vi "Test.vi"() -> ()   [LabVIEW 2015, in "LabSSH.lvlib"]
doc: "<License>This software is distributed under the BSD 3-Clause License. For the full license please see license.txt or visit www.labvolution.com/license</License>"
uses:
  LabSSH.lvlib
  Connection Info..cluster.ctl
  Password..cluster.ctl
  Private Public Key..cluster.ctl
  <vilib>/Utility/miscctls.llb/LVForegroundBackgroundColorsTypeDef.ctl
  connect_password.vi
  connect_key.vi
panel:
  in  "Connection Name":string
  in  "Close":bool
  in  "Connect":bool
  in  "Expected Response":string
  in  "Private_Public Key":T1
  in  "Connection Type":enum16{"Password", "Private Key"}(ring)
  out "Method Response":string
  in  "error in (no error)":errorcluster
  out "isSshConnected":bool
  in  "Password":T2
  in  "Connection Info.":T3={"Remote"="", "Username"="", "Port (22)"=22}
  out "Output":string
  # "http://www.labvolution.com/blog/"
  # "C:\\\\Working Folder\\\\ssh.git\\\\LabSSH\\\\raspberrypi_private_openssh.ppk"
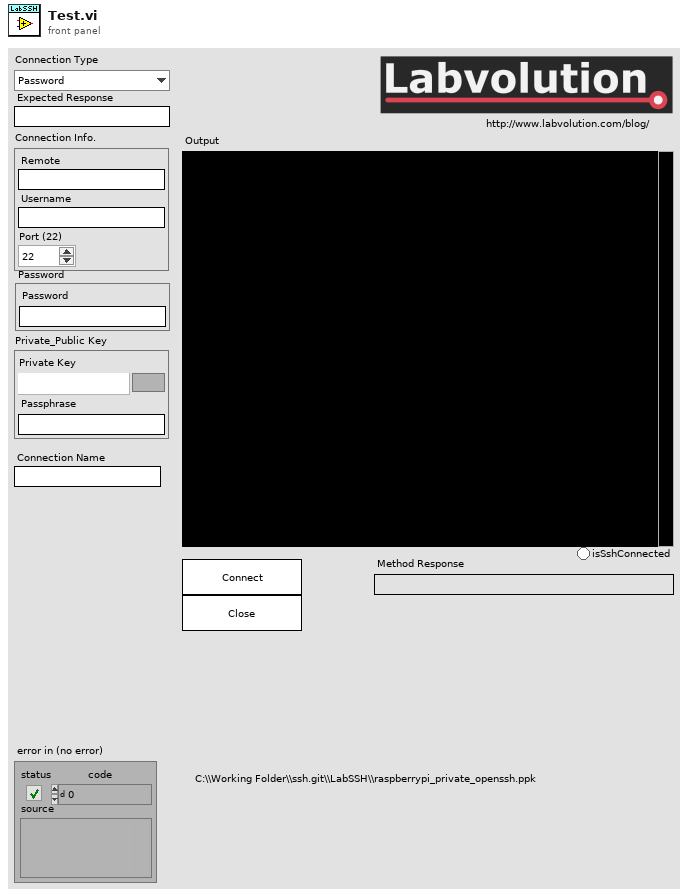
[diagram p1: front panel]
types:
  T1 = typedef "LabSSH.lvlib/Private Public Key..cluster.ctl" = cluster{"Private Key":path, "Passphrase":string}
  T2 = typedef "LabSSH.lvlib/Password..cluster.ctl" = cluster{"Password":string}
  T3 = typedef "LabSSH.lvlib/Connection Info..cluster.ctl" = cluster{"Remote":string, "Username":string, "Port (22)":i32}
  T4 = typedef "LVForegroundBackgroundColorsTypeDef.ctl" = cluster{"Foreground Color":u32, "Background Color":u32}
  T5 = enum32{"invalid app kind", "Development System", "Run Time System", "Student Edition", "Embedded LabVIEW", "Evaluation", "Custom"}
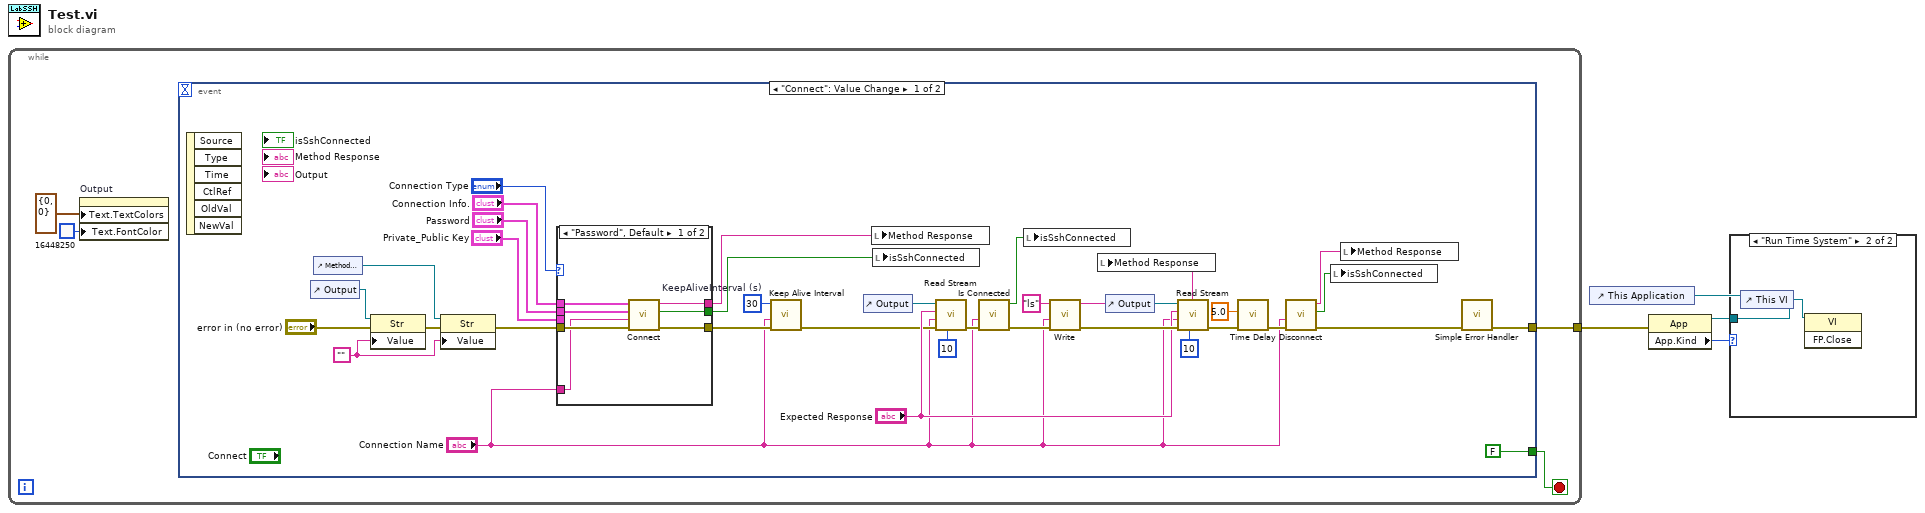
[diagram p0: block diagram]
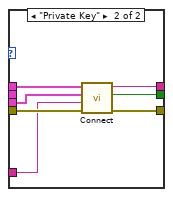
[diagram p2: hidden frame]
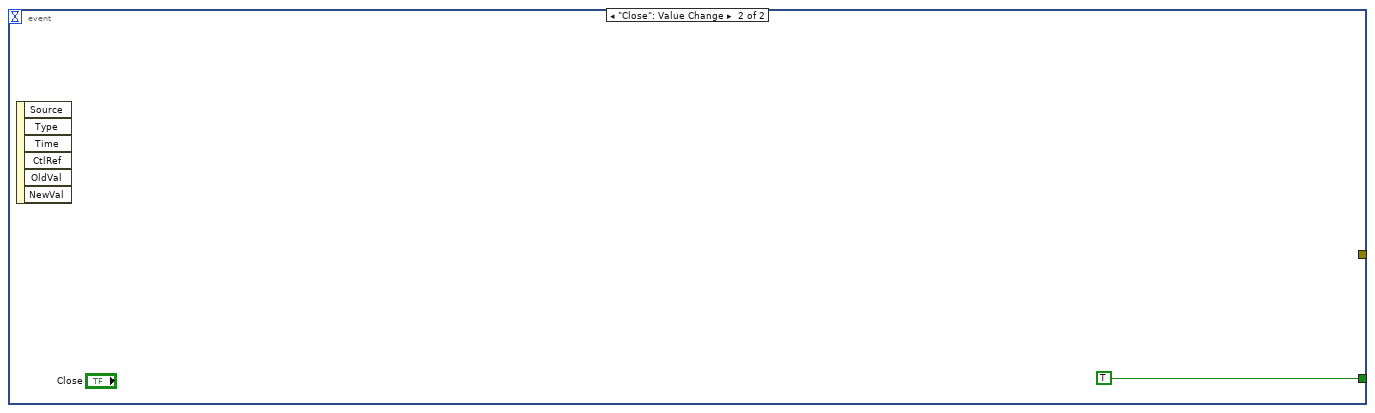
[diagram p3: hidden frame]
diagram:
  n1 = while {
    tunnel: [w5] -> w3
    stop <- w8 stop-if-true
    n2 = property on="Output" class="Str"("Text.TextColors"=T4 {"Foreground Color"=0, "Background Color"=0} ("Text.Colors"), "Text.FontColor"=u32 16448250 ("Text.Colors:BG Color")) -> ()  [unwired: 2 in, 2 out]
    n3 = event shown="[0] \"Connect\": Value Change" {
      selector: _ -> [_ _]
      dyn-events: _ -> [_ _]
      timeout: _ -> [_ _]
      tunnel: [FALSE TRUE] -> w8
      tunnel: [w15 _] -> w5
      event "Connect": Value Change {
        w11 = 30  # KeepAliveInterval (s)
        w23 = ""
        n4 = event-data() -> ()  [unwired: 1 in, 6 out]
        n5 = control-ref of="Output"() -> (w26:refnum<vi>)
        n6 = control-ref of="Method Response"() -> (w24:refnum<vi>)
        n7 = property class="Str"(reference=w26, error in="error in (no error)", "Value"=w23) -> (error out=w27:errorcluster)  [unwired: 1 out]
        n8 = property class="Str"(reference=w24, error in=w27, "Value"=w23) -> (error out=w25:errorcluster)  [unwired: 1 out]
        n9 = case shown="\"Password\", Default" "Connection Type" {
          tunnel: [w50 w55] -> w13
          tunnel: "Connection Info." -> [w49 w57]
          tunnel: "Password" -> [w48 _]
          tunnel: [w47 w54] -> w37
          tunnel: [w46 w53] -> w30
          tunnel: w25 -> [w45 w56]
          tunnel: "Private_Public Key" -> [_ w52]
          tunnel: "Connection Name" -> [w44 w51]
          frame "Password", Default {
            n10 = call-poly "Connect.vi"("error in (no error)"=w45, "Connection Name"=w44, "Password"=w48, "Connection Info."=w49) -> ("error out"=w50:errorcluster, "isSshConnected"=w47:bool, "Return String"=w46:string)  [unwired: 5 in]
          }
          frame "Private Key" {
            n11 = call-poly "Connect.vi"("error in (no error)"=w56, "Connection Name"=w51, "Private_Public Key"=w52, "Connection Info."=w57) -> ("error out"=w55:errorcluster, "isSshConnected"=w54:bool, "Return String"=w53:string)  [unwired: 5 in]
          }
        }
        n12 = call "Keep Alive Interval.vi"("error in (no error)"=w13, "Connection Name"="Connection Name", "KeepAliveInterval (s)"=w11) -> ("error out"=w14:errorcluster)  [unwired: 8 in]
        n13 = control-ref of="Output"() -> (w42:refnum<vi>)
        n14 = local write "Method Response"(w30) -> ()
        n15 = local write "isSshConnected"(w37) -> ()
        n16 = call "Read Stream.vi"("Timout (s)"=10, "error in (no error)"=w14, "Connection Name"="Connection Name", "Expected Response"="Expected Response", "Output ref"=w42) -> ("error out"=w38:errorcluster)  [unwired: 6 in]
        n17 = call "Is Connected.vi"("error in (no error)"=w38, "Connection Name"="Connection Name") -> ("error out"=w35:errorcluster, "isSshConnected"=w36:bool)  [unwired: 8 in]
        n18 = local write "isSshConnected"(w36) -> ()
        n19 = call "Write.vi"("error in (no error)"=w35, "Connection Name"="Connection Name", "Command"="ls") -> ("error out"=w31:errorcluster, "Return String"=w29:string)  [unwired: 7 in]
        n20 = local write "Method Response"(w29) -> ()
        n21 = control-ref of="Output"() -> (w33:refnum<vi>)
        n22 = call "Read Stream.vi"("Timout (s)"=10, "error in (no error)"=w31, "Connection Name"="Connection Name", "Expected Response"="Expected Response", "Output ref"=w33) -> ("error out"=w18:errorcluster)  [unwired: 6 in]
        n23 = call "Time Delay"("error in (no error)"=w18, "Delay Time (s)"=5.0) -> ("error out"=w17:errorcluster)  [unwired: 9 in]
        n24 = call "Disconnect.vi"("error in (no error)"=w17, "Connection Name"="Connection Name") -> ("error out"=w28:errorcluster, "isSshConnected"=w9:bool, "Return String"=w10:string)  [unwired: 7 in]
        n25 = local write "isSshConnected"(w9) -> ()
        n26 = local write "Method Response"(w10) -> ()
        n27 = call <vilib>:"Simple Error Handler.vi"("error in (no error)"=w28) -> ("error out"=w15:errorcluster)  [unwired: 4 in, 4 out]
      }
      event "Close": Value Change {
        n28 = event-data() -> ()  [unwired: 1 in, 6 out]
      }
    }
  }
  n29 = control-ref of="This Application"() -> (w4:refnum<vi>)
  n30 = property class="App"(reference=w4, error in=w3) -> (reference out=w1:refnum<vi>, "App.Kind"=w2:T5)  [unwired: 1 out]
  n31 = case shown="\"Run Time System\"" w2 {
    tunnel: w1 -> [_ _]
    frame "invalid app kind", Default {
    }
    frame "Run Time System" {
      n32 = control-ref of="This VI"() -> (w59:refnum<vi>)
      n33 = invoke class="VI" method="FP.Close"(reference=w59) -> ()  [unwired: 2 in, 3 out]
    }
  }
